vi "Process.vi"(8 "error in":errorcluster, 11 "Plugin in":refnum<class "StreamReader.lvclass">) -> (0 "error out":errorcluster, 3 "Plugin out":refnum<class "StreamReader.lvclass">)   [LabVIEW 2024, in "StreamReader.lvlib" / "StreamReader.lvclass"]
uses:
  StreamReader.lvclass
  C:/Program Files/National Instruments/LabVIEW 2024/vi.lib/FlexLogger/SDK/PluginSDK.lvlibp/PEFClasses/SDK/Plugin/Plugin.lvclass
  StreamReader.lvclass/StreamReader.ctl
  <vilib>/FlexLogger/SDK/PluginSDK.lvlibp/PEFClasses/SDK/Plugin/DataHelpers/Write 1D Wfm (DBL)_v2.vi
  <vilib>/FlexLogger/SDK/PluginSDK.lvlibp/PEFClasses/SDK/Plugin/Plugin.lvclass
  C:/Program Files/National Instruments/LabVIEW 2024/vi.lib/FlexLogger/SDK/PluginSDK.lvlibp/PEFClasses/SDK/Processing Element/Processing Element.lvclass
  C:/dev/niflexlogger-plugins/plugins/StreamReader/source/StreamReader.lvclass
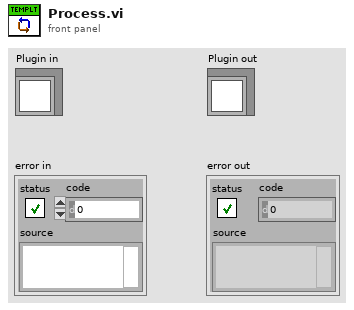
[diagram p1: front panel]
types:
  T1 = typedef "StreamReader.lvlib/StreamReader.lvclass/StreamReader Parameters.ctl" = cluster{"Reader URL":string, "Writer URL":string, "Timeout":i32, "Buffer Size":i32, "Reader endpoint":refnum<k21>, "Channel Names":string[]}
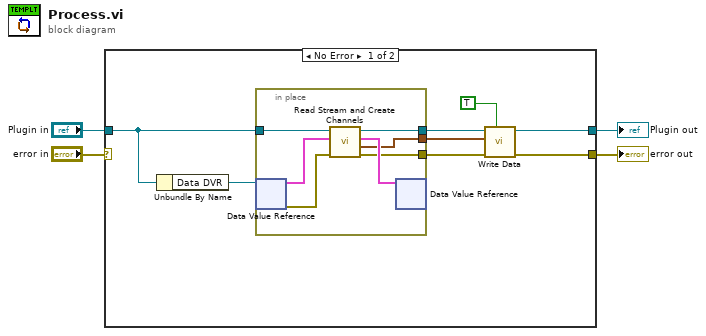
[diagram p0: block diagram]
diagram:
  n1 = case shown="No Error" "error in" {
    selector: "error in" -> [_ w20]
    tunnel: [w12 w21] -> w1
    tunnel: "Plugin in" -> [w6 w21]
    tunnel: [w5 w20] -> w2
    frame No Error {
      n2 = Unbundle By Name(w6) -> ("Data DVR"=w11:refnum<data-value>)
      n3 = in-place {
        in-place-border: w6 -> [w19]
        in-place-border: [w16] -> w10
        in-place-border: [w14] -> w9
        in-place-border: [w13] -> w8
        n4 = in-place-dvr #1(w11) -> (w18:T1, w17:errorcluster)
        n5 = call-dynamic "Read Stream and Create Channels.vi"("error in (no error)"=w17, "StreamReader Parameters in"=w18, "Plugin in"=w19) -> ("error out"=w14:errorcluster, "Array"=w13:waveform(dbl)[], "StreamReader Parameters out"=w15:T1, "Plugin out"=w16:refnum<class "StreamReader.lvclass">)  [unwired: 5 in]
        n6 = in-place-dvr #1(w15) -> ()  [unwired: 2 out]
      }
      n7 = call-poly <vilib>:"Write Data.vi"("Auto Calculate T0 (f)"=TRUE, "error in (no error)"=w9, "Data"=w8, "Plugin in"=w10) -> ("error out"=w5:errorcluster, "Plugin out"=w12:refnum<class "StreamReader.lvclass">)  [unwired: 6 in]
    }
    frame Error {
    }
  }
  "error out" <- w2
  "Plugin out" <- w1
